vi "MinimumJerkGenerateNext.vi"(10 "Target y":dbl, 11 "Target x":dbl) -> (2 "yt":dbl, 3 "xt":dbl)   [LabVIEW 2017, in "controllerLibrary.lvlib"]
uses:
  controllerLibrary.lvlib
  Controls/initial conditions control.ctl
  Controls/timer control.ctl
  Controls/tf control.ctl
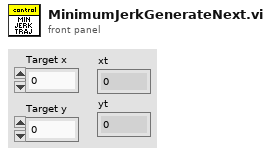
[diagram p1: front panel]
types:
  T1 = typedef "controllerLibrary.lvlib/tf control.ctl" = enum16{"get tf", "set tf"}
  T2 = typedef "controllerLibrary.lvlib/timer control.ctl" = enum16{"get time", "set time"}
  T3 = typedef "controllerLibrary.lvlib/initial conditions control.ctl" = enum16{"get", "set"}
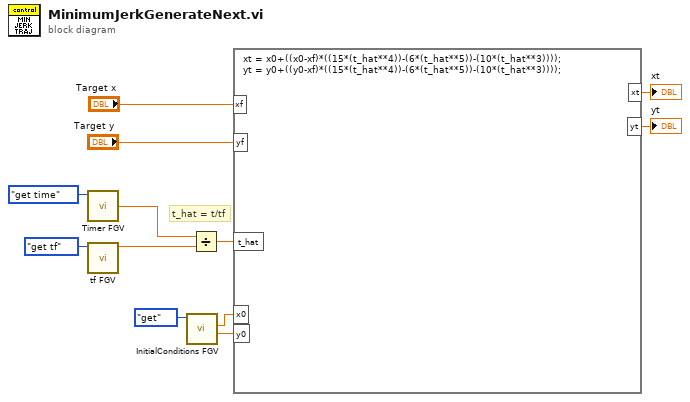
[diagram p0: block diagram]
diagram:
  # "t_hat = t/tf"
  n1 = call "Timer FGV.vi"("Enum"=timer_control."get time") -> ("Elapsed Time"=w2:dbl)  [unwired: 10 in]
  n2 = call "tf FGV.vi"("Enum"=tf_control."get tf") -> ("tf"=w1:dbl)  [unwired: 10 in]
  n3 = call "InitialConditions FGV.vi"("Enum"=initial_conditions_control."get") -> ("Y0"=w5:dbl, "X0"=w6:dbl)  [unwired: 9 in]
  n4 = Divide(x=w2, y=w1) -> (x/y=w10:dbl)
  n5 = formula code="xt = x0+((x0-xf)*((15*(t_hat**4))-(6*(t_hat**5))-(10*(t_hat**3))));\nyt = y0+((y0-xf)*((15*(t_hat**4))-(6*(t_hat**5))-(10*(t_hat**3))));"("t_hat"=w10, "x0"=w6, "y0"=w5, "xf"="Target x", "yf"="Target y") -> ("xt"=→"xt":dbl, "yt"=→"yt":dbl)
